vi "FlatToRichnixnet_grpc_WriteFrameRequest.vi"(5 "OutputClusterType":T1, 11 "InputCluster":T4) -> (3 "OutputCluster":T1)   [LabVIEW 2025, in "grpc-xnet_client.lvlib"]
uses:
  nixnet_grpc_WriteFrameRequest_Flat.ctl
  nidevice_grpc_Session_Flat.ctl
  nixnet_grpc_FrameBufferRequest_Flat.ctl
  nixnet_grpc_FrameRequest_Flat.ctl
  nixnet_grpc_FrameType.ctl
  nixnet_grpc_FrameFlags.ctl
  nixnet_grpc_EnetFrameRequest_Flat.ctl
  nixnet_grpc_EnetFrameType.ctl
  nixnet_grpc_EnetFlags.ctl
  nixnet_grpc_TimeOut.ctl
  nixnet_grpc_WriteFrameRequest.ctl
  nixnet_grpc_WriteFrameRequest_timeout_enum/nixnet_grpc_WriteFrameRequest_timeout_enum.lvclass
  nidevice_grpc_Session.ctl
  nixnet_grpc_FrameBufferRequest.ctl
  nixnet_grpc_FrameBufferRequest_frame/nixnet_grpc_FrameBufferRequest_frame.lvclass
  grpc-xnet_client.lvlib
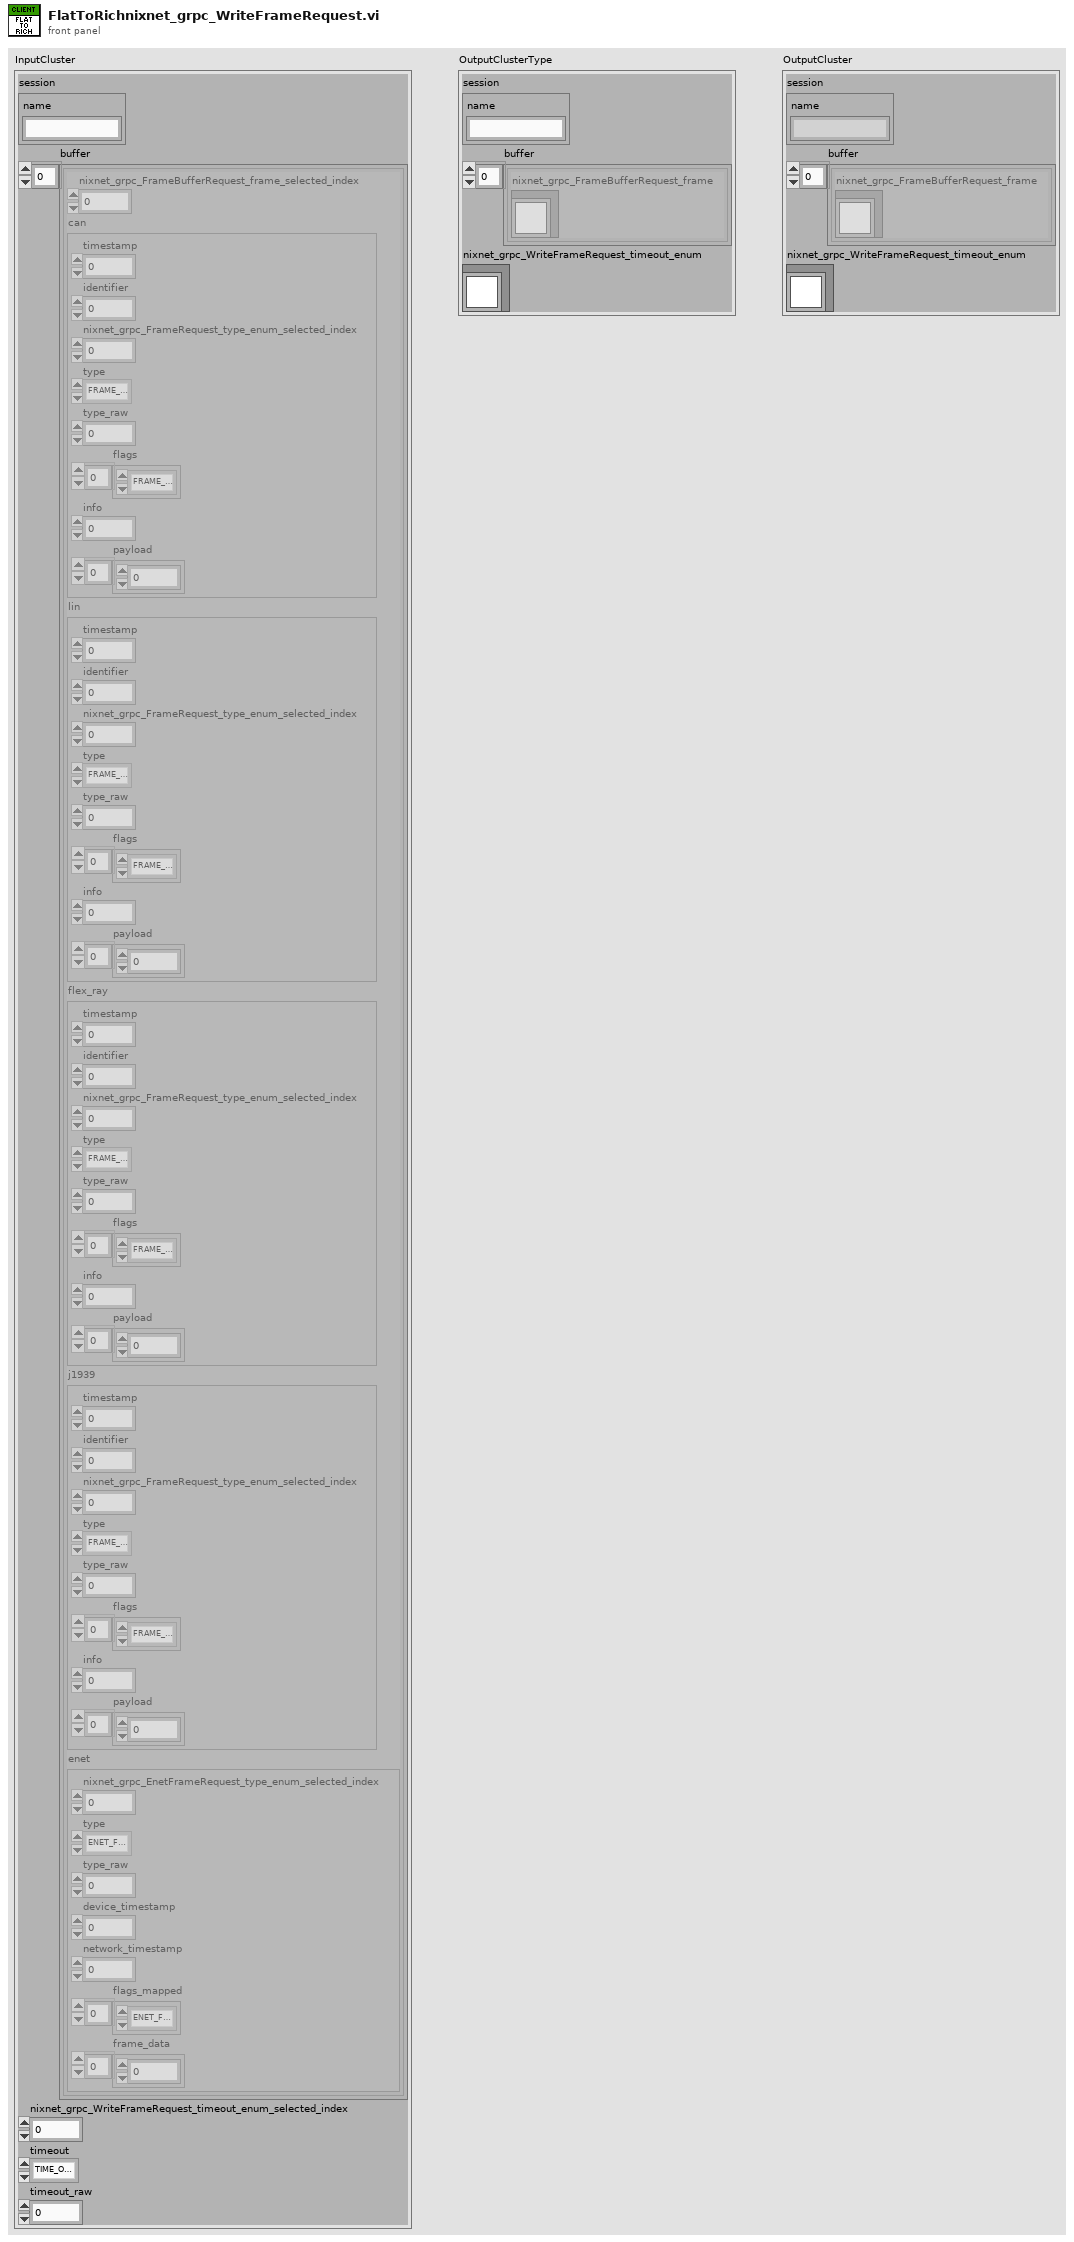
[diagram p1: front panel]
types:
  T1 = typedef "grpc-xnet_client.lvlib/nixnet_grpc_WriteFrameRequest.ctl" = cluster{"session":T2, "buffer":T3[], "nixnet_grpc_WriteFrameRequest_timeout_enum":refnum<class "nixnet_grpc_WriteFrameRequest_timeout_enum.lvclass">}
  T2 = typedef "grpc-xnet_client.lvlib/nidevice_grpc_Session.ctl" = cluster{"name":string}
  T3 = typedef "grpc-xnet_client.lvlib/nixnet_grpc_FrameBufferRequest.ctl" = cluster{"nixnet_grpc_FrameBufferRequest_frame":refnum<class "nixnet_grpc_FrameBufferRequest_frame.lvclass">}
  T4 = typedef "grpc-xnet_client.lvlib/nixnet_grpc_WriteFrameRequest_Flat.ctl" = cluster{"session":T5, "buffer":T6[], "nixnet_grpc_WriteFrameRequest_timeout_enum_selected_index":i32, "timeout":T13, "timeout_raw":dbl}
  T5 = typedef "grpc-xnet_client.lvlib/nidevice_grpc_Session_Flat.ctl" = cluster{"name":string}
  T6 = typedef "grpc-xnet_client.lvlib/nixnet_grpc_FrameBufferRequest_Flat.ctl" = cluster{"nixnet_grpc_FrameBufferRequest_frame_selected_index":i32, "can":T7, "lin":T7, "flex_ray":T7, "j1939":T7, "enet":T10}
  T7 = typedef "grpc-xnet_client.lvlib/nixnet_grpc_FrameRequest_Flat.ctl" = cluster{"timestamp":u64, "identifier":u32, "nixnet_grpc_FrameRequest_type_enum_selected_index":i32, "type":T8, "type_raw":u32, "flags":T9[], "info":u32, "payload":u8[]}
  T8 = typedef "grpc-xnet_client.lvlib/nixnet_grpc_FrameType.ctl" = enum32{"FRAME_TYPE_CAN_DATA", "FRAME_TYPE_CAN_REMOTE", "FRAME_TYPE_CAN_BUS_ERROR", "FRAME_TYPE_CAN20_DATA", "FRAME_TYPE_CANFD_DATA", "FRAME_TYPE_CANFDBRS_DATA", "FRAME_TYPE_FLEX_RAY_DATA", "FRAME_TYPE_FLEX_RAY_NULL", "FRAME_TYPE_FLEX_RAY_SYMBOL", "FRAME_TYPE_LIN_DATA", "FRAME_TYPE_LIN_BUS_ERROR", "FRAME_TYPE_LIN_NO_RESPONSE", "FRAME_TYPE_J1939_DATA", "FRAME_TYPE_SPECIAL_DELAY", "FRAME_TYPE_SPECIAL_LOG_TRIGGER", "FRAME_TYPE_SPECIAL_START_TRIGGER"}
  T9 = typedef "grpc-xnet_client.lvlib/nixnet_grpc_FrameFlags.ctl" = enum32{"FRAME_FLAGS_UNSPECIFIED", "FRAME_FLAGS_FLEX_RAY_STARTUP", "FRAME_FLAGS_FLEX_RAY_SYNC", "FRAME_FLAGS_FLEX_RAY_PREAMBLE", "FRAME_FLAGS_FLEX_RAY_CH_A", "FRAME_FLAGS_FLEX_RAY_CH_B", "FRAME_FLAGS_LIN_EVENT_SLOT", "FRAME_FLAGS_TRANSMIT_ECHO"}
  T10 = typedef "grpc-xnet_client.lvlib/nixnet_grpc_EnetFrameRequest_Flat.ctl" = cluster{"nixnet_grpc_EnetFrameRequest_type_enum_selected_index":i32, "type":T11, "type_raw":u32, "device_timestamp":u64, "network_timestamp":u64, "flags_mapped":T12[], "frame_data":u8[]}
  T11 = typedef "grpc-xnet_client.lvlib/nixnet_grpc_EnetFrameType.ctl" = enum32{"ENET_FRAME_TYPE_DATA", "ENET_FRAME_TYPE_DELAY", "ENET_FRAME_TYPE_FUTURE_TIME_WAIT"}
  T12 = typedef "grpc-xnet_client.lvlib/nixnet_grpc_EnetFlags.ctl" = enum32{"ENET_FLAGS_UNSPECIFIED", "ENET_FLAGS_TRANSMIT", "ENET_FLAGS_RECEIVE", "ENET_FLAGS_NETWORK_SYNCED", "ENET_FLAGS_ERROR"}
  T13 = typedef "grpc-xnet_client.lvlib/nixnet_grpc_TimeOut.ctl" = enum32{"TIME_OUT_NONE", "TIME_OUT_INFINITE"}
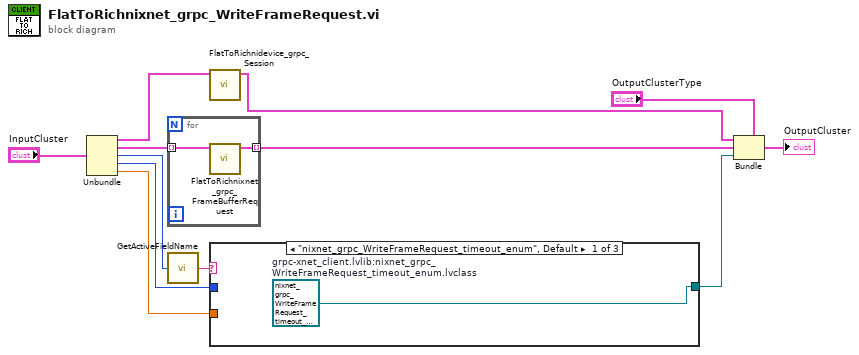
[diagram p0: block diagram]
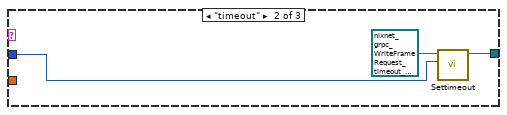
[diagram p2: hidden frame]
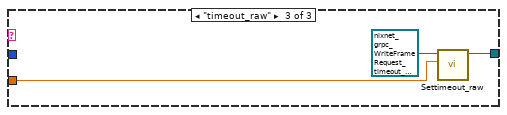
[diagram p3: hidden frame]
diagram:
  n1 = Unbundle "Unbundle"("InputCluster") -> ("session"=w9:T5, "buffer"=w7:T6[], "nixnet_grpc_WriteFrameRequest_timeout_enum_selected_index"=w5:i32, "timeout"=w2:T13, "timeout_raw"=w1:dbl)
  n2 = for {
    tunnel: w7 -> [w14] mode=indexing
    tunnel: [w13] -> w6 mode=indexing
    n3 = call "FlatToRichnixnet_grpc_FrameBufferRequest.vi"("InputCluster"=w14) -> ("OutputCluster"=w13:T3)  [unwired: 10 in]
  }
  n4 = call "GetActiveFieldName.vi"("protobuf index"=w5) -> ("oneof field name"=w4:string)
  n5 = call "FlatToRichnidevice_grpc_Session.vi"("InputCluster"=w9) -> ("OutputCluster"=w8:T2)  [unwired: 10 in]
  n6 = case "nixnet_grpc_WriteFrameRequest_timeout_enum" shown="\"nixnet_grpc_WriteFrameRequest_timeout_enum\", Default" w4 {
    tunnel: [w15 w17 w20] -> w3
    tunnel: w2 -> [_ w18 _]
    tunnel: w1 -> [_ _ w21]
    frame "nixnet_grpc_WriteFrameRequest_timeout_enum", Default {
      w15 = refnum<class "nixnet_grpc_WriteFrameRequest_timeout_enum.lvclass"> refnum  # grpc-xnet_client.lvlib:nixnet_grpc_WriteFrameRequest_timeout_enum.lvclass
    }
    frame "timeout" {
      n7 = call "Settimeout.vi"("Set_Val"=w18, "OneOfTemplate in"=refnum<class "nixnet_grpc_WriteFrameRequest_timeout_enum.lvclass"> refnum) -> ("OneOfTemplate out"=w17:refnum<class "nixnet_grpc_WriteFrameRequest_timeout_enum.lvclass">)  [unwired: 8 in, 1 out]
    }
    frame "timeout_raw" {
      n8 = call "Settimeout_raw.vi"("Set_Val"=w21, "OneOfTemplate in"=refnum<class "nixnet_grpc_WriteFrameRequest_timeout_enum.lvclass"> refnum) -> ("OneOfTemplate out"=w20:refnum<class "nixnet_grpc_WriteFrameRequest_timeout_enum.lvclass">)  [unwired: 8 in, 1 out]
    }
  }
  n9 = Bundle "Bundle"(cluster="OutputClusterType", "session"=w8, "buffer"=w6, "nixnet_grpc_WriteFrameRequest_timeout_enum"=w3) -> (→"OutputCluster":T1)
